vi "Init Notifiers.vi"(8 "error in (no error)":errorcluster, 11 "Transport in":refnum<class "Transport.lvclass">) -> (0 "error out":errorcluster, 3 "Transport out":refnum<class "Transport.lvclass">)   [LabVIEW 2019, in "Transport.lvclass"]
uses:
  Transport.lvclass
  Transport.lvclass/Transport.ctl
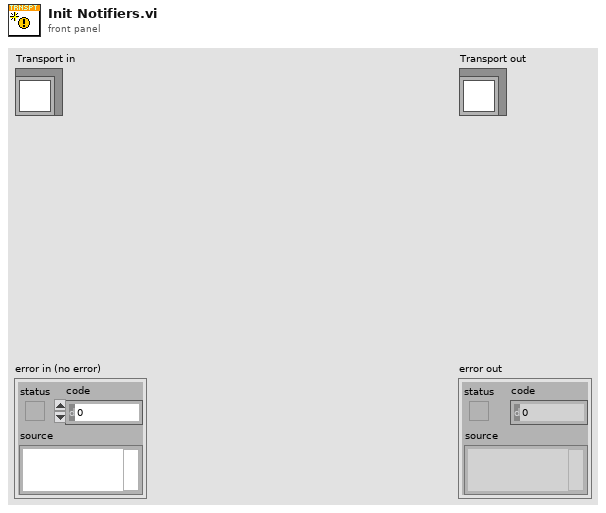
[diagram p1: front panel]
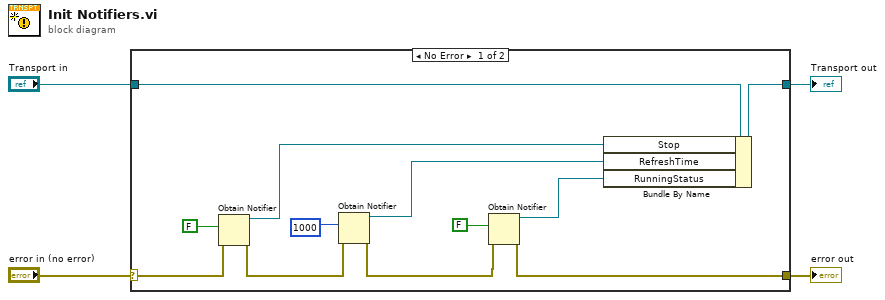
[diagram p0: block diagram]
diagram:
  n1 = case shown="No Error" "error in (no error)" {
    selector: "error in (no error)" -> [w13 w17]
    tunnel: [w5 w17] -> w3
    tunnel: [w15 w18] -> w1
    tunnel: "Transport in" -> [w16 w18]
    frame No Error {
      n2 = Obtain Notifier(notification data type=FALSE, error in (no error)=w13) -> (notifier out=w8:refnum<notifier>, error out=w7:errorcluster)  [unwired: 2 in, 1 out]
      n3 = Obtain Notifier(notification data type=u32 1000, error in (no error)=w7) -> (notifier out=w10:refnum<notifier>, error out=w6:errorcluster)  [unwired: 2 in, 1 out]
      n4 = Obtain Notifier(notification data type=FALSE, error in (no error)=w6) -> (notifier out=w9:refnum<notifier>, error out=w5:errorcluster)  [unwired: 2 in, 1 out]
      n5 = Bundle By Name(cluster=w16, "Stop"=w8, "RefreshTime"=w10, "RunningStatus"=w9) -> (w15:refnum<class "Transport.lvclass">)
    }
    frame Error {
    }
  }
  "error out" <- w3
  "Transport out" <- w1
